vi "Normalize.vi"(1 "Current Angle":dbl, 2 "Initial Angle":dbl) -> (0 "Normalized Angle":dbl)   [LabVIEW 2015]
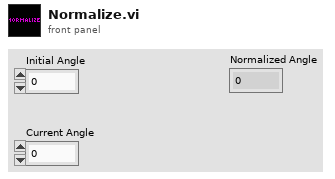
[diagram p1: front panel]
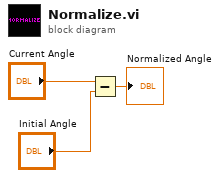
[diagram p0: block diagram]
diagram:
  n1 = Subtract(x="Current Angle", y="Initial Angle") -> (x-y=→"Normalized Angle":dbl)
